vi "Remove piece.vi"(10 "Square":T1={"File"=enum."a", "Rank"=enum."4"}, 11 "Board in":refnum<class "Board.lvclass">) -> (1 "Removed piece":refnum<class "Piece.lvclass">, 2 "Square occupied?":bool, 3 "Board out":refnum<class "Board.lvclass">)   [LabVIEW 2015, in "Chesslib.lvlib" / "Board.lvclass"]
uses:
  Board.lvclass
  typedef/Square.ctl
  typedef/File.ctl
  typedef/Rank.ctl
  Pieces/Piece/Piece.lvclass
  Board.lvclass/Board.ctl
  Chesslib.lvlib
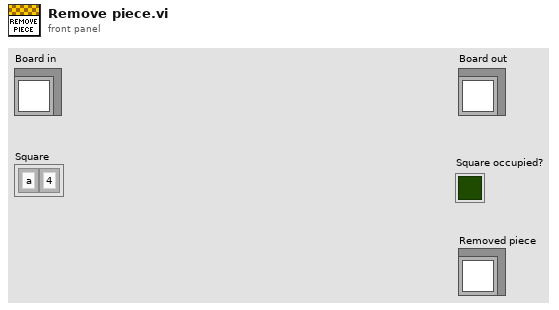
[diagram p1: front panel]
types:
  T1 = typedef "Chesslib.lvlib/Square.ctl" = cluster{"File":T2, "Rank":T3}
  T2 = typedef "Chesslib.lvlib/File.ctl" = enum16{"a", "b", "c", "d", "e", "f", "g", "h"}
  T3 = typedef "Chesslib.lvlib/Rank.ctl" = enum16{"1", "2", "3", "4", "5", "6", "7", "8"}
  T4 = cluster{"Occupied":bool, "Piece":refnum<class "Piece.lvclass">}[]
  T5 = cluster{"Occupied":bool, "Piece":refnum<class "Piece.lvclass">}
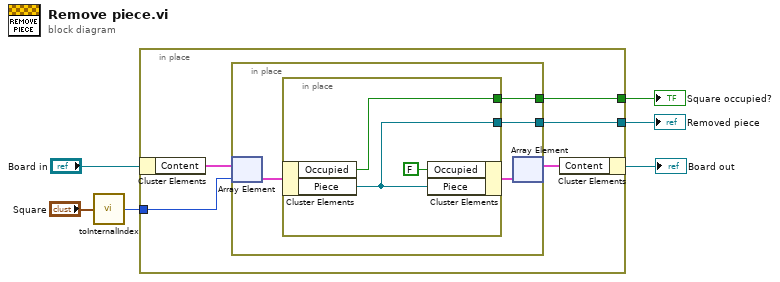
[diagram p0: block diagram]
diagram:
  n1 = call "toInternalIndex.vi"("Square"="Square") -> ("Internal index"=w3:u8)
  n2 = in-place "In Place Element Structure" {
    in-place-border: w3 -> [w9]
    in-place-border: [w8] -> w1
    in-place-border: [w7] -> w2
    n3 = in-place-cluster #1("Board in") -> ("Content"=w11:T4)
    n4 = in-place {
      in-place-border: [w13] -> w8
      in-place-border: [w12] -> w7
      n5 = in-place-array #2(w11, w9) -> (w15:T5)
      n6 = in-place {
        in-place-border: [w18] -> w13
        in-place-border: [w17] -> w12
        n7 = in-place-cluster #3(w15) -> ("Occupied"=w18:bool, "Piece"=w17:refnum<class "Piece.lvclass">)
        n8 = in-place-cluster #3("Occupied"=FALSE, "Piece"=w17) -> (w14:T5)
      }
      n9 = in-place-array #2(w14) -> (w10:T4)  [unwired: 1 out]
    }
    n10 = in-place-cluster #1("Content"=w10) -> (→"Board out":refnum<class "Board.lvclass">)
  }
  "Removed piece" <- w2
  "Square occupied?" <- w1
